vi "TW_BuildJSON.vi"(11 "Tag":T1) -> (2 "JSON":string, 3 "URL":string)   [LabVIEW 2019]
uses:
  TW_Ctrl.ctl
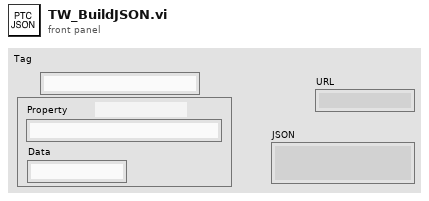
[diagram p1: front panel]
types:
  T1 = typedef "TW_Ctrl.ctl" = cluster{"Thing":string, "Property":string, "Type":string, "Data":string}
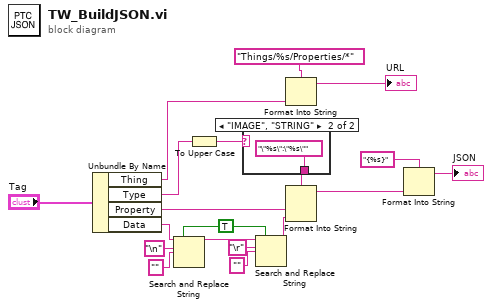
[diagram p0: block diagram]
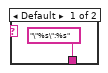
[diagram p2: hidden frame]
diagram:
  w14 = TRUE ("replace all? (F)")
  n1 = Unbundle By Name("Tag") -> ("Thing"=w19:string, "Type"=w5:string, "Property"=w3:string, "Data"=w7:string)
  n2 = Search and Replace String(replace all?=w14, input string=w7, search string="\n", replace string="" ("replace string (\"\")")) -> (result string=w12:string)  [unwired: 4 in, 3 out]
  n3 = To Upper Case(1:w5) -> (0:w6:string)
  n4 = case shown="\"IMAGE\", \"STRING\"" w6 {
    tunnel: ["\"%s\":%s" ("format string") "\"%s\":\"%s\"" ("format string")] -> w4
    frame Default {
    }
    frame "IMAGE", "STRING" {
    }
  }
  n5 = Search and Replace String(replace all?=w14, input string=w12, search string="\r", replace string="" ("replace string (\"\")")) -> (result string=w13:string)  [unwired: 4 in, 3 out]
  n6 = Format Into String(format string="Things/%s/Properties/*", w19) -> (resulting string=→"URL":string)  [unwired: 2 in, 1 out]
  n7 = Format Into String(format string=w4, w3, w13) -> (resulting string=w16:string)  [unwired: 2 in, 1 out]
  n8 = Format Into String(format string="{%s}", w16) -> (resulting string=→"JSON":string)  [unwired: 2 in, 1 out]
